vi "SendData.vi"(8 "error in":errorcluster, 11 "Input Array":string[][](array[string])) -> (0 "error out":errorcluster)   [LabVIEW 2014]
uses:
  Controls/CMWQCluster.ctl
  Controls/CMWQEnum.ctl
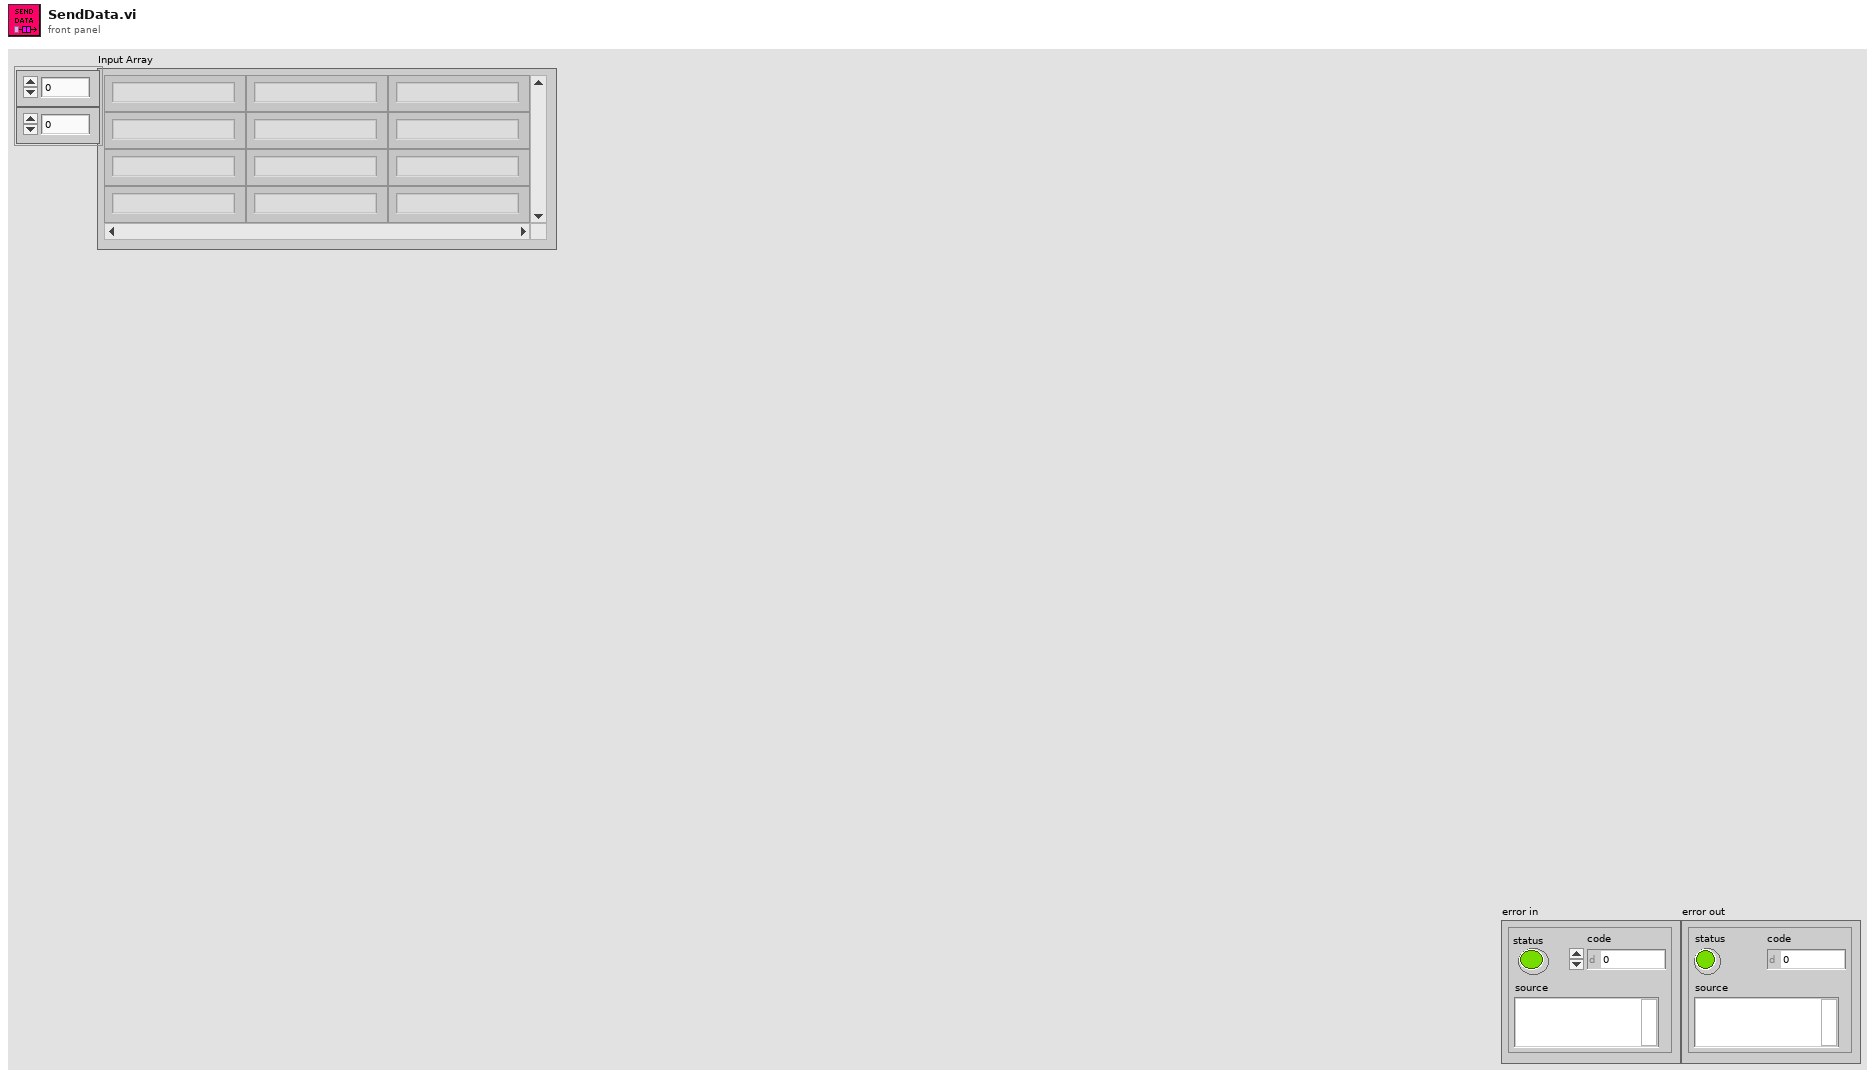
[diagram p1: front panel]
types:
  T1 = typedef "CMWQCluster.ctl" = cluster{"Variant":variant, "Enum":T2}
  T2 = typedef "CMWQEnum.ctl" = enum16{"Initialise", "Acquire", "Stop"}
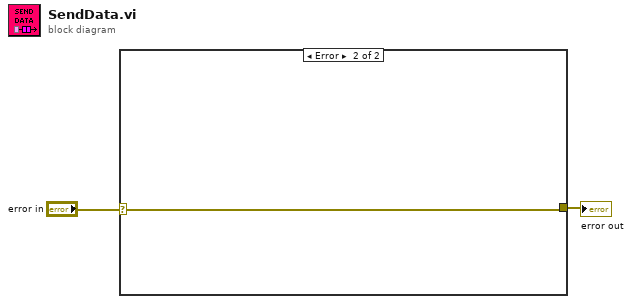
[diagram p0: block diagram]
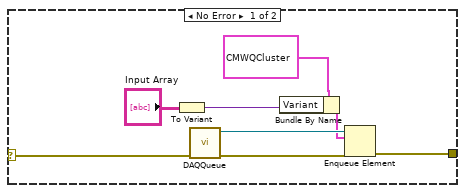
[diagram p2: hidden frame]
diagram:
  n1 = case shown="Error" "error in" {
    selector: "error in" -> [w3 w11]
    tunnel: [w5 w11] -> w2
    frame No Error {
      n2 = To Variant(anything="Input Array") -> (Variant=w6:variant)
      n3 = call "DAQQueue.vi"("error in"=w3) -> ("error out"=w10:errorcluster, "queue out"=w9:refnum<queue>)  [unwired: 8 in]
      n4 = Bundle By Name(cluster=T1 {"Variant"=variant, "Enum"=enum."Initialise"}, "Variant"=w6) -> (w7:T1)
      n5 = Enqueue Element(queue=w9, element=w7, error in (no error)=w10) -> (error out=w5:errorcluster)  [unwired: 1 in, 2 out]
    }
    frame Error {
    }
  }
  "error out" <- w2
